vi "Date.vi"(10 "UTC format":bool) -> (2 "date/time string":string)   [LabVIEW 2019]
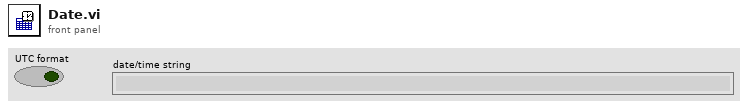
[diagram p1: front panel]
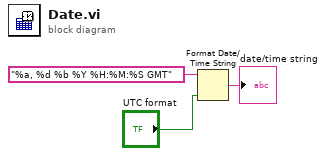
[diagram p0: block diagram]
diagram:
  n1 = Format Date/Time String(time format string (%c)="%a, %d %b %Y %H:%M:%S GMT", UTC format="UTC format") -> (date/time string=→"date/time string":string)  [unwired: 1 in]
